vi "host.vi"() -> ()   [LabVIEW 2010]
uses:
  <vilib>/rvi/interface/nirviReadWriteControl/nirviReadWriteControl.xnode
  <vilib>/rvi/interface/nirviMethod/nirviMethod.xnode
  <vilib>/rvi/interface/nirviCloseFPGA/nirviCloseFPGA.xnode
  <vilib>/rvi/interface/nirviOpenFPGA/nirviOpenFPGA.xnode
  <vilib>/userDefined/High Color/nirio_resource_hc.ctl
  <vilib>/Utility/error.llb/Error Cluster From Error Code.vi
  <vilib>/rvi/errors/niLvFpgaWhatHappensToTopLevelVI.ctl
  <vilib>/rvi/interface/common/niFpgaNodeNameForErrorReporting.ctl
  <vilib>/rvi/errors/niLvFpgaAdjustHostInterfaceError.vi
  NiFpgaLv.dll
  <vilib>/FPGAPlugInAG/sbRIO-9642/niLvFpga_Abort_sbRIO-9642.vi
  LIA_FPGA.vi
  <vilib>/RVI Host/nirviSupport.llb/nirviErrorClusterFromErrorCode.vi
  <vilib>/FPGAPlugInAG/sbRIO-9642/niLvFpga_Close_sbRIO-9642.vi
panel:
  out "Actual Sampling Frequency":dbl
  in  "input range of 9205":dbl=10.0
  in  "resource name":T1 caption="RIO Device"
  in  "Sampling Frequency":dbl=50000.0 min=1000.0 max=250000.0
  in  "stop":bool
  out "degree":dbl
  out "r":dbl
  out "y":dbl
  out "x":dbl
  out "f":dbl format="%.2g"
  in  "dec2":i16=1
  in  "nominal freq":dbl=1000.0 min=500.0 max=125000.0
  in  "dec1":i16=1000
  in  "stages":i8=1 min=1 max=2
  in  "decimation":i16=1000
  # "Sampling Frequency"
  # "CIC First Decimation"
  # "CIC Second Decimation"
  # "MA Stages"
  # "MA Decimation"
  # "PLL Nominal Frequency"
  # "PLL Frequency Output"
  # "LIA Output"
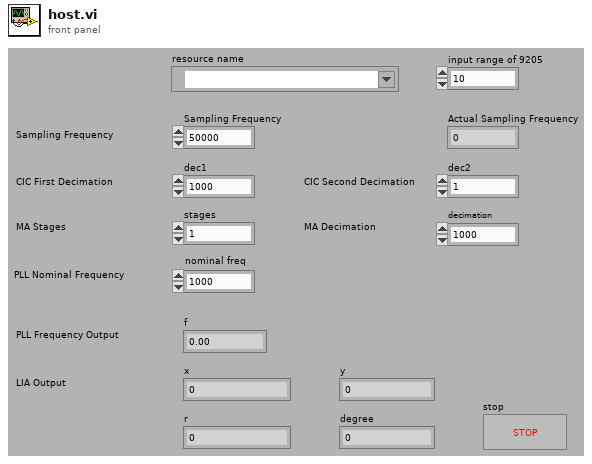
[diagram p1: front panel]
types:
  T1 = typedef "nirio_resource_hc.ctl" = tag
  T2 = typedef "niFpgaNodeNameForErrorReporting.ctl" = enum16{"Open FPGA VI Reference", "Read/Write Control", "Invoke Method: Abort", "Invoke Method: Acknowledge IRQ", "Invoke Method: Download", "Invoke Method: FIFO.Configure", "Invoke Method: FIFO.Read", "Invoke Method: FIFO.Start", "Invoke Method: FIFO.Stop", "Invoke Method: FIFO.Write", "Invoke Method: Reset", "Invoke Method: Run", "Invoke Method: Wait on IRQ", "Close FPGA VI Reference"}
  T3 = typedef "niLvFpgaWhatHappensToTopLevelVI.ctl" = enum16{"top level VI scripted behind XNode", "top level VI inlined behind XNode"}
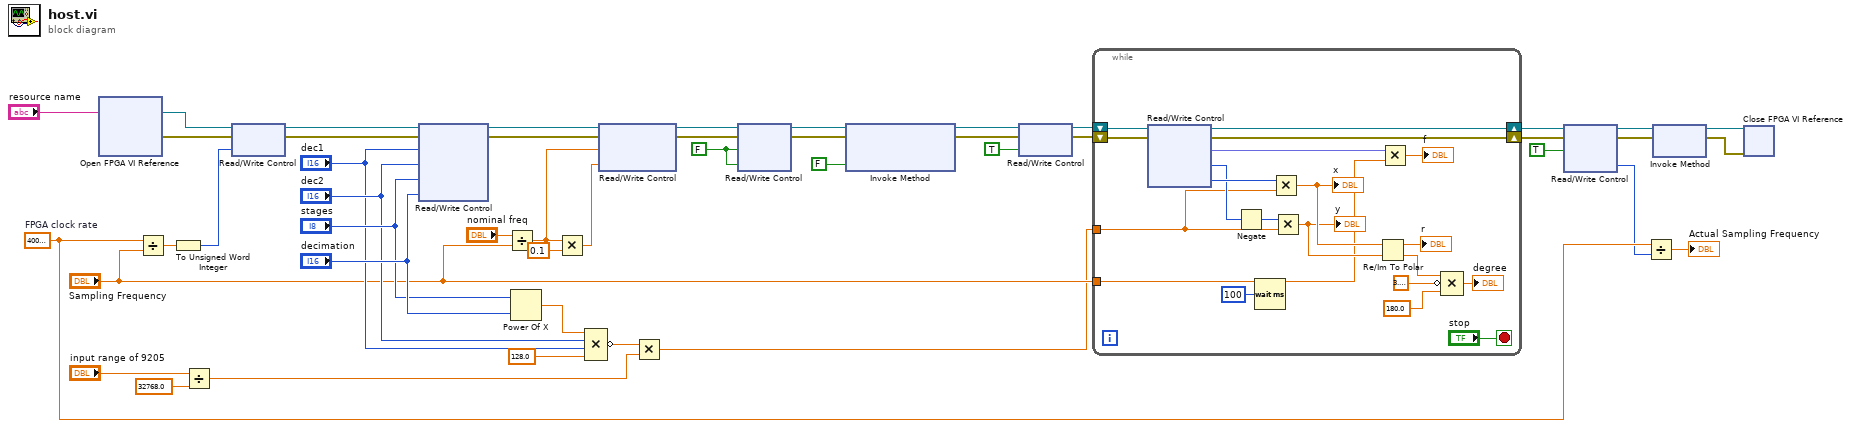
[diagram p0: block diagram]
diagram:
  w3 = 40000000.0  # FPGA clock rate
  w24 = FALSE ("start")
  n1 = xnode "Open FPGA VI Reference"("resource name"="resource name") -> ("FPGA VI Reference Out"=w10:refnum<k20>, "error out"=w9:errorcluster)  [unwired: 1 in]
  n2 = Divide(x=w3, y="Sampling Frequency") -> (x/y=w17:dbl)
  n3 = To Unsigned Word Integer(number=w17) -> (unsigned 16bit integer=w16:u16)
  n4 = Divide(x="input range of 9205", y=32768.0) -> (x/y=w4:dbl)
  n5 = xnode "Read/Write Control"("FPGA VI Reference In"=w10, "error in"=w9, "Period"=w16) -> ("FPGA VI Reference Out"=w19:refnum<k20>, "error out"=w18:errorcluster)
  n6 = xnode "Read/Write Control"("FPGA VI Reference In"=w19, "error in"=w18, "dec1"="dec1", "dec2"="dec2", "stages"="stages", "decimation"="decimation") -> ("FPGA VI Reference Out"=w46:refnum<k20>, "error out"=w45:errorcluster)
  n7 = Divide(x="nominal freq", y="Sampling Frequency") -> (x/y=w13:dbl)
  n8 = Power Of X(1:"decimation", 2:"stages") -> (0:w41:dbl)
  n9 = Multiply(x=w13, y=0.1) -> (x*y=w11:dbl)
  n10 = Compound Arithmetic op=MULTIPLY(w41, "dec2", "dec1", 128.0) -> (invert w37:dbl)
  n11 = xnode "Read/Write Control"("FPGA VI Reference In"=w46, "error in"=w45, "nominal freq"=w13, "K"=w11) -> ("FPGA VI Reference Out"=w28:refnum<k20>, "error out"=w27:errorcluster)
  n12 = Multiply(x=w37, y=w4) -> (x*y=w5:dbl)
  n13 = xnode "Read/Write Control"("FPGA VI Reference In"=w28, "error in"=w27, "start"=w24, "stop"=w24) -> ("FPGA VI Reference Out"=w26:refnum<k20>, "error out"=w25:errorcluster)
  n14 = xnode "Invoke Method"("FPGA VI Reference In"=w26, "error in"=w25, "Wait Until Done (F)"=FALSE) -> ("FPGA VI Reference Out"=w33:refnum<k20>, "error out"=w31:errorcluster)
  n15 = xnode "Read/Write Control"("FPGA VI Reference In"=w33, "error in"=w31, "start"=TRUE) -> ("FPGA VI Reference Out"=w32:refnum<k20>, "error out"=w30:errorcluster)
  n16 = while {
    shift-right: [w61] -> w36
    shift-left: w32 -> [w66]
    shift-right: [w60] -> w35
    shift-left: w30 -> [w65]
    tunnel: w5 -> [w62]
    tunnel: "Sampling Frequency" -> [w49]
    stop <- "stop" stop-if-true
    n17 = xnode "Read/Write Control"("FPGA VI Reference In"=w66, "error in"=w65) -> ("FPGA VI Reference Out"=w61:refnum<k20>, "error out"=w60:errorcluster, "f"=w50:fxp<+/-,32,0>, "channelQ"=w63:i64, "channelI"=w64:i64)
    n18 = Negate(x=w63) -> (-x=w47:i64)
    n19 = Wait (ms)(milliseconds to wait=u32 100) -> ()  [unwired: 1 out]
    n20 = Multiply(x=w64, y=w62) -> (x*y=w59:dbl)
    "x" <- w59
    n21 = Multiply(x=w47, y=w62) -> (x*y=w58:dbl)
    "y" <- w58
    n22 = Re/Im To Polar(2:w58, 3:w59) -> (0:w56:dbl, 1:→"r":dbl)
    n23 = Multiply(x=w50, y=w49) -> (x*y=→"f":dbl)
    n24 = Compound Arithmetic op=MULTIPLY(w56, invert 3.141592653589793, 180.0 ("value")) -> (→"degree":dbl)
  }
  n25 = xnode "Read/Write Control"("FPGA VI Reference In"=w36, "error in"=w35, "stop"=TRUE) -> ("FPGA VI Reference Out"=w23:refnum<k20>, "error out"=w22:errorcluster, "ticks"=w2:u16)
  n26 = Divide(x=w3, y=w2) -> (x/y=→"Actual Sampling Frequency":dbl)
  n27 = xnode "Invoke Method"("FPGA VI Reference In"=w23, "error in"=w22) -> ("FPGA VI Reference Out"=w21:refnum<k20>, "error out"=w20:errorcluster)
  n28 = xnode "Close FPGA VI Reference"("FPGA VI Reference In"=w21, "error in"=w20) -> ()  [unwired: 1 out]
